vi "Read Main Path.vi"(8 "error in (no error)":errorcluster, 11 "Error Logger in":refnum<class "Error Logger.lvclass">) -> (0 "error out":errorcluster, 2 "Main Path":path, 3 "Error Logger out":refnum<class "Error Logger.lvclass">)   [LabVIEW 2012, in "Error Logger.lvclass"]
uses:
  Error Logger.lvclass
  Error Logger.lvclass/Error Logger.ctl
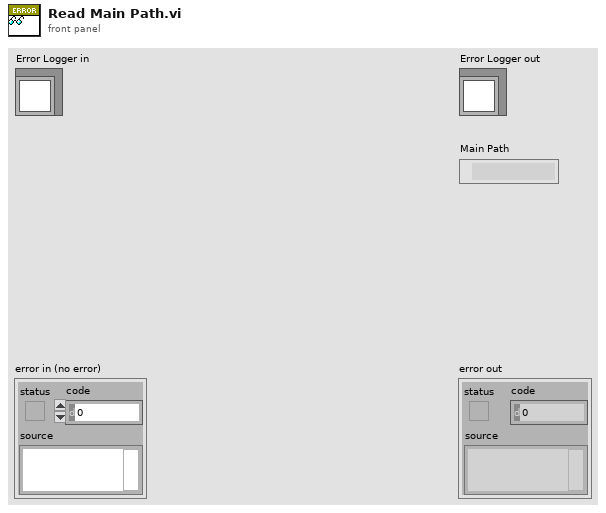
[diagram p1: front panel]
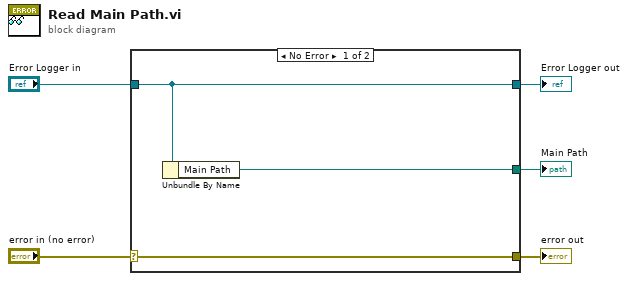
[diagram p0: block diagram]
diagram:
  n1 = case shown="No Error" "error in (no error)" {
    selector: "error in (no error)" -> [w8 w9]
    tunnel: [w8 w9] -> w4
    tunnel: [w7 w10] -> w2
    tunnel: "Error Logger in" -> [w7 w10]
    tunnel: [w6 _] -> w1
    frame No Error {
      n2 = Unbundle By Name(w7) -> ("Main Path"=w6:path)
    }
    frame Error {
    }
  }
  "error out" <- w4
  "Error Logger out" <- w2
  "Main Path" <- w1
